vi "Create CAN Outgoing Section.vi"(8 "error in (no error)":errorcluster, 11 "Parent Ref in":T1 format="%.0x") -> (0 "error out":errorcluster, 3 "Parent Ref out":T1 format="%.0x")   [LabVIEW 2023, in "J1939 Addon Shared.lvlib"]
uses:
  J1939 Addon Shared.lvlib
  <vilib>/NI VeriStand/Custom Device API/Custom Device Item Ref.ctl
  Constants.vi
  <vilib>/NI/NI VeriStand Advanced SysDef API/SysDef API/Advanced System Definition.lvlib
  <vilib>/NI VeriStand/Custom Device API/Custom Device API.lvlib
panel:
  # "OUTPUTS"
  # "INPUTS"
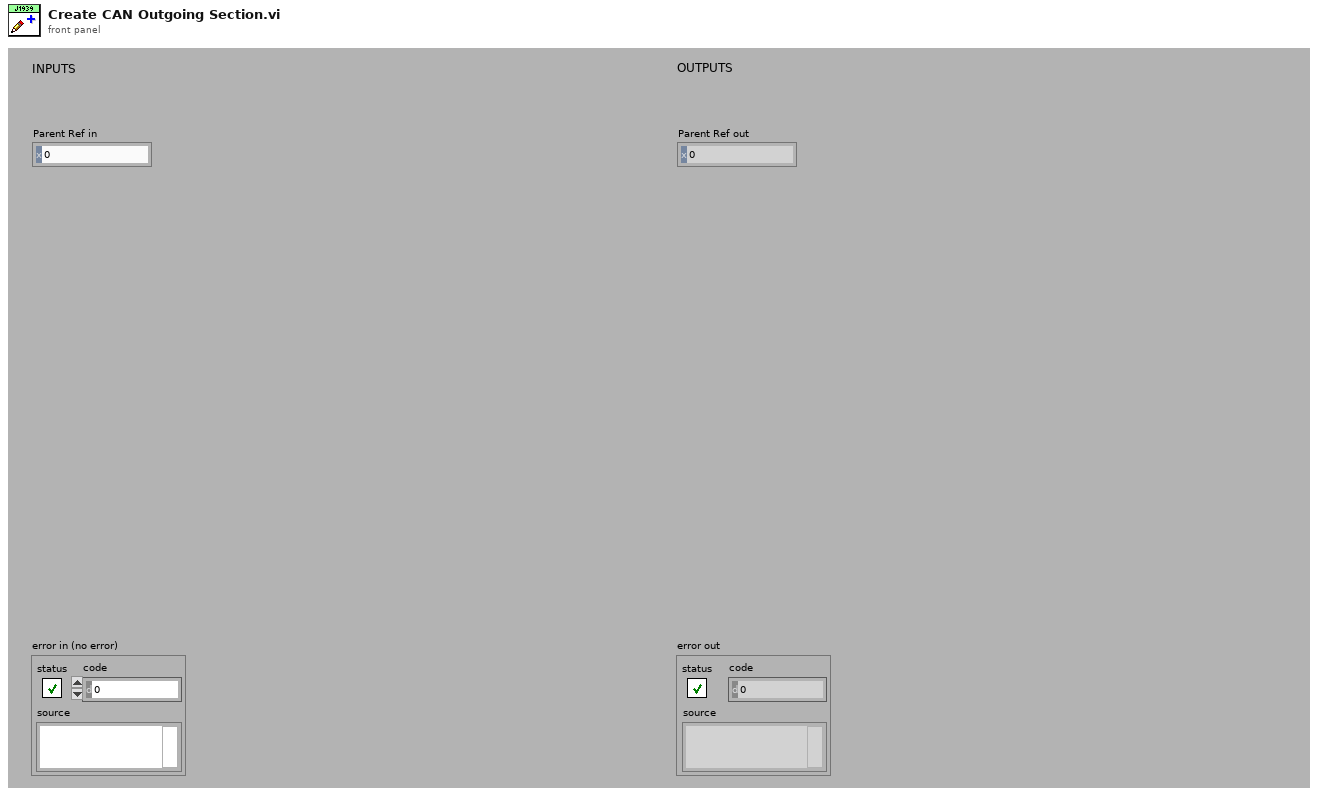
[diagram p1: front panel]
types:
  T1 = typedef "Custom Device API.lvlib/Custom Device Item Ref.ctl" = u64
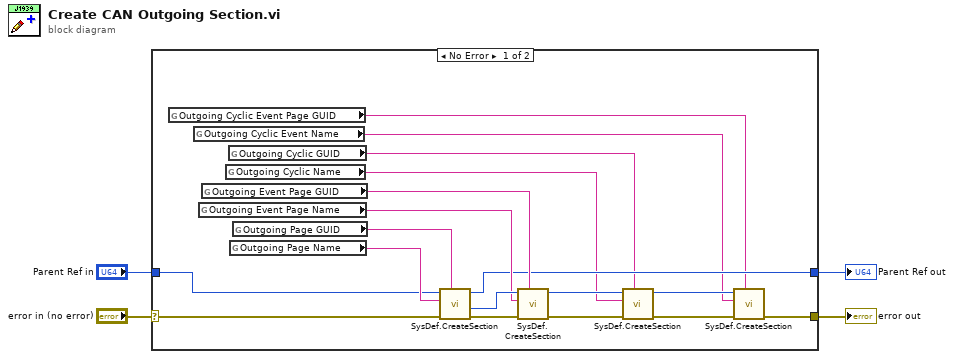
[diagram p0: block diagram]
diagram:
  n1 = case shown="No Error" "error in (no error)" {
    selector: "error in (no error)" -> [w16 w24]
    tunnel: [w8 w24] -> w3
    tunnel: "Parent Ref in" -> [w15 w23]
    tunnel: [w14 w23] -> w1
    frame No Error {
      n2 = global read "Constants.vi" "Outgoing Cyclic Event Page GUID"() -> (w6:string)
      n3 = global read "Constants.vi" "Outgoing Cyclic Event Name"() -> (w5:string)
      n4 = global read "Constants.vi" "Outgoing Event Page Name"() -> (w17:string)
      n5 = global read "Constants.vi" "Outgoing Event Page GUID"() -> (w18:string)
      n6 = global read "Constants.vi" "Outgoing Cyclic Name"() -> (w10:string)
      n7 = global read "Constants.vi" "Outgoing Cyclic GUID"() -> (w11:string)
      n8 = global read "Constants.vi" "Outgoing Page Name"() -> (w19:string)
      n9 = global read "Constants.vi" "Outgoing Page GUID"() -> (w20:string)
      n10 = call <vilib>:"SysDef.CreateSection.vi"("GUID"=w20, "error in (no error)"=w16, "Name"=w19, "nodeID"=w15) -> ("error out"=w22:errorcluster, "New NodeID"=w21:u64, "nodeID out"=w14:u64)  [unwired: 4 in, 1 out]
      n11 = call <vilib>:"SysDef.CreateSection.vi"("GUID"=w18, "error in (no error)"=w22, "Name"=w17, "nodeID"=w21) -> ("error out"=w13:errorcluster, "nodeID out"=w12:u64)  [unwired: 4 in, 2 out]
      n12 = call <vilib>:"SysDef.CreateSection.vi"("GUID"=w11, "error in (no error)"=w13, "Name"=w10, "nodeID"=w12) -> ("error out"=w9:errorcluster, "nodeID out"=w7:u64)  [unwired: 4 in, 2 out]
      n13 = call <vilib>:"SysDef.CreateSection.vi"("GUID"=w6, "error in (no error)"=w9, "Name"=w5, "nodeID"=w7) -> ("error out"=w8:errorcluster)  [unwired: 4 in, 3 out]
    }
    frame Error {
    }
  }
  "error out" <- w3
  "Parent Ref out" <- w1
